vi "GetErrorInfo.vi"(8 "error in (no error)":errorcluster, 11 "ErrorNumber":i32=1) -> (0 "error out":errorcluster, 1 "restart?":bool, 2 "severity":T2(ring), 3 "Error{}":T1)   [LabVIEW 2009]
doc: "This vi returns the error message of the input error number\n\n12/21/2010 1.0.0 jyg\n- initial release"
uses:
  NEO VI Example/data/icsneo40.dll
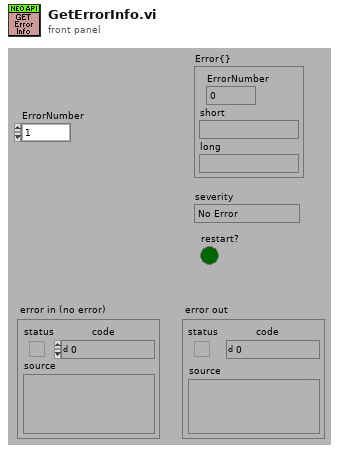
[diagram p1: front panel]
types:
  T1 = cluster{"ErrorNumber":i32, "short":string, "long":string}
  T2 = enum16{"No Error", "Critical", "Important", "Warning", "Unknown"}
  T3 = cluster{"ErrorNumber":i32, "trimmed string":string, "trimmed string":string}
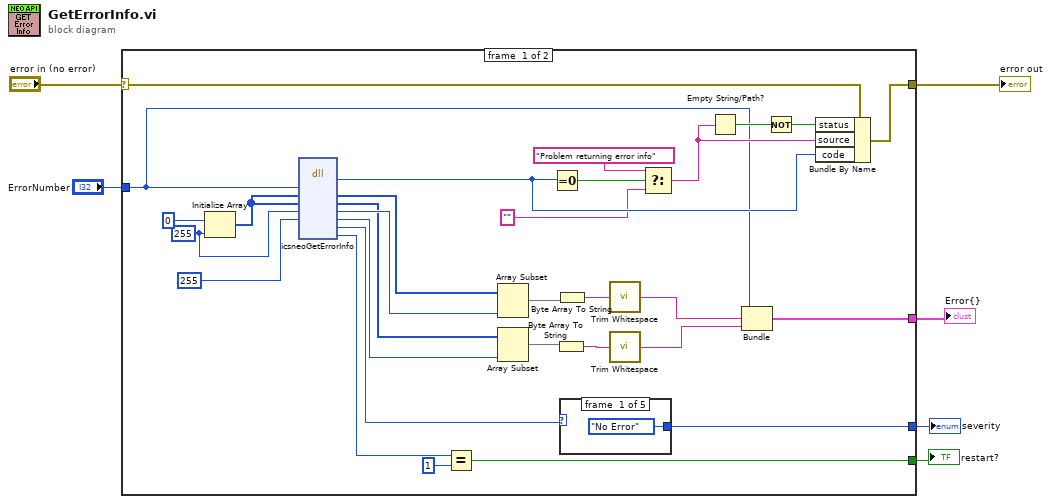
[diagram p0: block diagram]
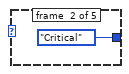
[diagram p2: hidden frame]
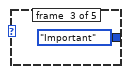
[diagram p3: hidden frame]
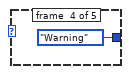
[diagram p4: hidden frame]
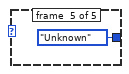
[diagram p5: hidden frame]
diagram:
  n1 = case shown="No Error" "error in (no error)" {
    selector: "error in (no error)" -> [w32 w42]
    tunnel: [w33 w42] -> w6
    tunnel: "ErrorNumber" -> [w9 _]
    tunnel: [w19 _] -> w4
    tunnel: [w16 _] -> w3
    tunnel: [w8 _] -> w1
    frame #0 {
      w26 = 255 ("dimension size")
      n2 = Initialize Array(i8 0, w26) -> (w27:i8[])
      n3 = dll-call lib="C:/WINDOWS/system32/icsneo40.dll" fn="icsneoGetErrorInfo"("ErrorNumber"=w9, "ErrorShort"=w27, "ErrorLong"=w27, "ErrorShortLength"=w26, "ErrorLongLength"=255 ("dimension size")) -> ("return type"=w31:i32, "ErrorShort"=w24:i8[], "ErrorLong"=w22:i8[], "ErrorShortLength"=w23:i32, "ErrorLongLength"=w21:i32, "Severity"=w20:i32, "Restart"=w18:i32)  [unwired: 4 in, 4 out]
      n4 = Equal?(x=w18, y=1) -> (x = y?=w16:bool)
      n5 = Array Subset(array=w24, length=w23) -> (w15:i8[])  [unwired: 1 in]
      n6 = Array Subset(array=w22, length=w21) -> (w14:i8[])  [unwired: 1 in]
      n7 = Equal To 0?(x=w31) -> (x = 0?=w30:bool)
      n8 = Byte Array To String(unsigned byte array=w14) -> (string=w12:string)
      n9 = Byte Array To String(unsigned byte array=w15) -> (string=w13:string)
      n10 = case shown="0, Default" w20 {
        tunnel: [T2."No Error" T2."Critical" T2."Important" T2."Warning" T2."Unknown"] -> w19
        frame #0 {
        }
        frame #1 {
        }
        frame #2 {
        }
        frame #3 {
        }
        frame #4 {
        }
      }
      n11 = call <vilib>:"Trim Whitespace.vi"("string"=w13) -> ("trimmed string"=w11:string)  [unwired: 1 in]
      n12 = call <vilib>:"Trim Whitespace.vi"("string"=w12) -> ("trimmed string"=w10:string)  [unwired: 1 in]
      n13 = Select(t="Problem returning error info", s=w30, f="") -> (s? t:f=w29:string)
      n14 = Empty String/Path?(string/path=w29) -> (empty?=w35:bool)
      n15 = Bundle("ErrorNumber"=w9, "trimmed string"=w11, "trimmed string"=w10) -> (w8:T3)  [unwired: 1 out]
      n16 = Not(x=w35) -> (.not. x?=w34:bool)
      n17 = Bundle By Name(cluster=w32, "status"=w34, "source"=w29, "code"=w31) -> (w33:errorcluster)
    }
    frame #1 {
    }
  }
  "error out" <- w6
  "severity" <- w4
  "restart?" <- w3
  "Error{}" <- w1
